vi "Main - Hover.vi"() -> ()   [LabVIEW 2017]
doc: "The myRIO Project template acquires acceleration data from the onboard accelerometer and displays the changes of acceleration values in a waveform chart."
uses:
  <vilib>/myRIO/Instrument Drivers/Onboard IO/PWM/typedefs/PWM Reference.ctl
  <vilib>/myRIO/Common/Instrument Driver Framework/Utilities/typedefs/myRIO Generic Hardware Reference.ctl
  <vilib>/myRIO/Common/Instrument Driver Framework/Utilities/typedefs/Hardware Version Enum.ctl
  <vilib>/myRIO/Common/Instrument Driver Framework/Utilities/typedefs/myRIO v1.0 Reference.ctl
  <vilib>/myRIO/Common/Instrument Driver Framework/Utilities/typedefs/Generic FPGA Reference.ctl
  <vilib>/myRIO/Common/Instrument Driver Framework/myRIO v1.0/PWM/typedefs/PWM Channels Enum.ctl
  <vilib>/myRIO/Instrument Drivers/Onboard IO/PWM/typedefs/PWM Configuration.ctl
  <vilib>/userdefined/High Color/nirio_resource_hc.ctl
  <vilib>/myRIO/Instrument Drivers/Onboard Devices/Accelerometer/typedefs/Accelerometer Reference.ctl
  <vilib>/myRIO/Common/Instrument Driver Framework/myRIO v1.0/Accelerometer/typedefs/Accelerometer Channels List.ctl
  <vilib>/myRIO/Common/Instrument Driver Framework/myRIO v1.0/Accelerometer/typedefs/Accelerometer Channels Enum.ctl
  <vilib>/myRIO/Common/Instrument Driver Framework/Utilities/vis/Is FPGA Ref Available.vi
  <vilib>/myRIO/Common/Instrument Driver Framework/myRIO v1.0/PWM/vis/myRIO v1.1 Open PWM.vi
  <vilib>/myRIO/Instrument Drivers/Onboard IO/PWM/vis/Set Duty Cycle and Frequency.vi
  <vilib>/myRIO/Common/Instrument Driver Framework/myRIO v1.0/Accelerometer/vis/myRIO v1.1 Open Accelerometer.vi
  <vilib>/myRIO/Instrument Drivers/Onboard Devices/Accelerometer/vis/Read.vi
  <vilib>/myRIO/Common/Instrument Driver Framework/Utilities/vis/Validate Channels.vi
  <vilib>/myRIO/Common/Instrument Driver Framework/myRIO v1.0/PWM/vis/myRIO v1.0 Reserve PWM.vi
  <vilib>/myRIO/Common/Instrument Driver Framework/myRIO v1.0/Accelerometer/vis/myRIO v1.0 Reserve Accelerometer.vi
  <vilib>/myRIO/Common/Instrument Driver Framework/myRIO v1.0/UART/vis/myRIO v1.0 Close UART.vi
  <vilib>/myRIO/Common/Instrument Driver Framework/myRIO v1.0/PWM/vis/myRIO v1.0 Build MUX Configuration PWM.vi
  <vilib>/myRIO/Common/Instrument Driver Framework/myRIO v1.0/Resource Manager/vis/myRIO v1.0 Reserve Channel List.vi
  <vilib>/myRIO/Common/Instrument Driver Framework/myRIO v1.0/Accelerometer/vis/myRIO v1.0 Build MUX Configuration Accelerometer.vi
  <vilib>/myRIO/Common/Instrument Driver Framework/myRIO v1.0/Resource Manager/vis/myRIO v1.0 Create Configuration List.vi
  <vilib>/myRIO/Common/Instrument Driver Framework/myRIO v1.0/Resource Manager/vis/myRIO v1.0 Reserve Channel.vi
  <vilib>/myRIO/Common/Instrument Driver Framework/myRIO v1.0/Resource Manager/vis/myRIO v1.0 Unreserve Channel.vi
  <vilib>/myRIO/Common/Instrument Driver Framework/myRIO v1.0/Resource Manager/vis/myRIO v1.0 Build Mutex Name.vi
  <vilib>/Utility/VariantDataType/GetNumericInfo.vi
  <vilib>/Utility/error.llb/Error Cluster From Error Code.vi
  <vilib>/myRIO/Common/Instrument Driver Framework/myRIO v1.0/myRIO v1.1 Open.vi
  <vilib>/myRIO/Common/Instrument Driver Framework/Utilities/vis/IO Manager.vi
  <vilib>/myRIO/Common/Instrument Driver Framework/Utilities/vis/Configuration Manager.vi
  <vilib>/myRIO/Common/Instrument Driver Framework/myRIO v1.0/Resource Manager/vis/myRIO v1.0 Configure IO.vi
  <vilib>/myRIO/Common/Instrument Driver Framework/myRIO v1.0/myRIO v1.0 Close.vi
  <vilib>/myRIO/Common/Instrument Driver Framework/myRIO v1.0/PWM/vis/myRIO v1.0 Write PWM.vi
  <vilib>/myRIO/Common/Instrument Driver Framework/myRIO v1.0/Accelerometer/vis/myRIO v1.0 Get Scaling Constant Accelerometer.vi
  <vilib>/myRIO/Common/Instrument Driver Framework/myRIO v1.0/Accelerometer/vis/myRIO v1.0 Read Accelerometer.vi
  <vilib>/myRIO/Common/Instrument Driver Framework/Utilities/vis/FPGA Ref Manager.vi
  <vilib>/myRIO/Common/Instrument Driver Framework/myRIO v1.0/myRIO v1.0 Reset FPGA.vi
  <vilib>/myRIO/Common/Instrument Driver Framework/myRIO v1.0/IRQ/vis/myRIO v1.0 IRQ Info FGV.vi
  <vilib>/myRIO/Common/Instrument Driver Framework/myRIO v1.0/IRQ/vis/myRIO v1.0 Timer IRQ Info FGV.vi
  <vilib>/myRIO/Common/Instrument Driver Framework/myRIO v1.0/IRQ/vis/myRIO v1.0 ISR Agent.vi
  <vilib>/myRIO/Express VI/Onboard IO/PWM/PWM Express VI.xnode
  <vilib>/myRIO/Instrument Drivers/Onboard IO/PWM/vis/myRIO PWM Open.xnode
  <vilib>/myRIO/Express VI/Onboard Devices/Accelerometer/Accelerometer Express VI.xnode
  <vilib>/myRIO/Instrument Drivers/Onboard Devices/Accelerometer/vis/myRIO Accelerometer Open.xnode
  <vilib>/myRIO/Instrument Drivers/Utilities/Utilities.lvlib
  <vilib>/myRIO/Instrument Drivers/Onboard Devices/Accelerometer/Accelerometer.lvlib
  <vilib>/myRIO/Instrument Drivers/Onboard IO/PWM/PWM.lvlib
panel:
  in  "[ESC]":bool
  out "X rot rate":i16
  out "Y rot rate":i16
  out "Z rot rate":i16
  out "Angular rate [LSB/sec]":cluster{dbl, dbl, dbl}(graph)
  out "Angular displacement [LSB]":T1(graph)
  out "X displacement":dbl format="%#_5g"
  out "Y displacement":dbl format="%#_5g"
  out "Z displacement":dbl format="%#_5g"
  in  "reset integrator":bool
  out "X acc":i16
  out "Y acc":i16
  out "Z acc":i16
  out "Temp":i16
  out "Linear Acceleration [LSB/sec^2]":cluster{i16, i16, i16}(graph)
  in  "Duty Cycle MCC2 : Faixa de operação":dbl
  out "Acceleration 2":T2(graph)
  in  "Brushless controller Duty Cycle":dbl(slide)=0.05 scale=0.05..0.1 scale format="%#_6f"
  in  "Controle sentido M2":bool
  in  "Duty Cycle MCC1 : Faixa de operação":dbl
  in  "Ligar (StandBy)":bool
  in  "Controle sentido M1":bool
  in  "Stop":bool
  # "Overview: The myRIO Project template acquires acceleration data from the onboard accelerometer and displays the changes of acceleration values in a waveform chart.\nInstructions:\n1. Check the myRIO target IP address in the project and make sure the target IP address is correct. \n2. Run this VI."
  # "2"
  # "1"
  # "2"
  # "1"
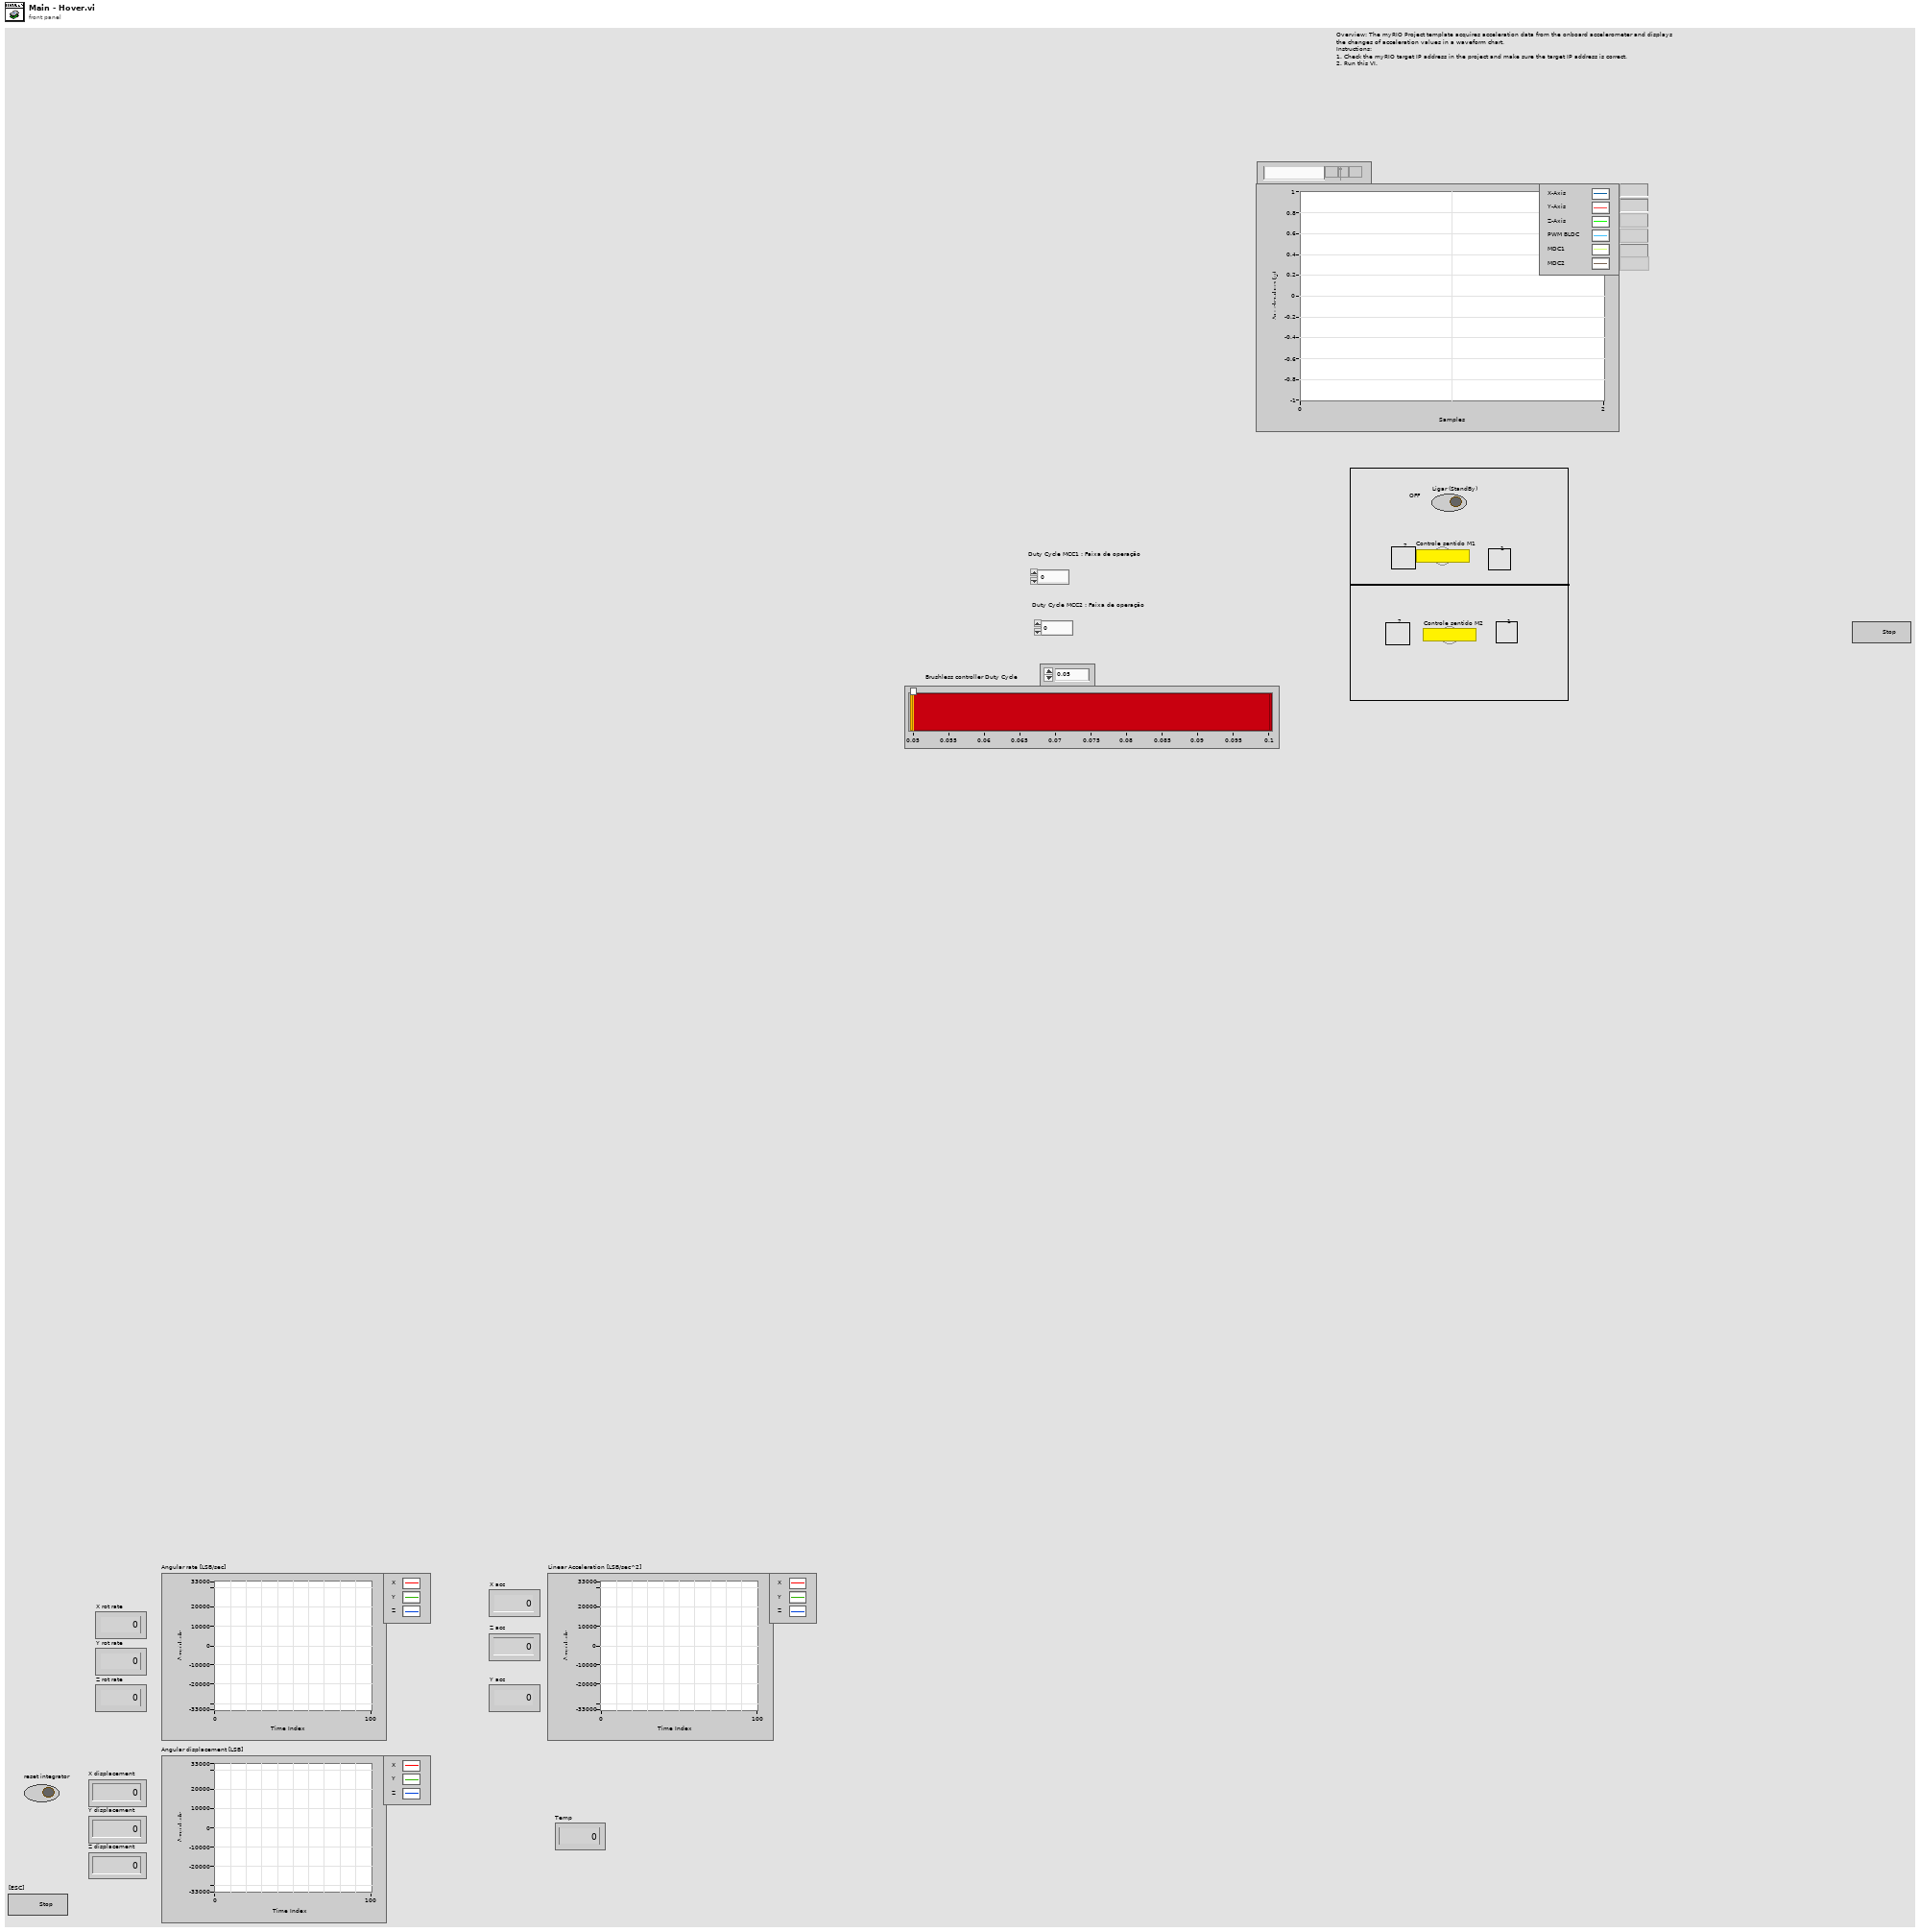
[diagram p1: front panel]
types:
  T1 = cluster{"integral x(t)":dbl, "integral x(t)":dbl, "integral x(t)":dbl}
  T2 = cluster{"X-Axis":dbl, "Y-Axis":dbl, "Z-Axis":dbl, "Brushless controller Duty Cycle":dbl, "\nDuty Cycle MCC1 : Faixa de operação":dbl, "\nDuty Cycle MCC2 : Faixa de operação ":dbl}
  T3 = typedef "PWM.lvlib/PWM Reference.ctl" = cluster{"myRIO Reference":T4, "PWM Channels Enum":T8, "PWM Configuration":T9}
  T4 = typedef "myRIO Generic Hardware Reference.ctl" = cluster{"myRIO Model":T5, "myRIO Hardware Reference":T6}
  T5 = typedef "Hardware Version Enum.ctl" = enum16{"Unknown", "myRIO-1900", "myRIO-1950", "roboRIO", "NI ELVIS RIO CM"}
  T6 = typedef "myRIO v1.0 Reference.ctl" = cluster{"Generic FPGA Reference":T7, "Allow multiple opens":bool}
  T7 = typedef "Generic FPGA Reference.ctl" = refnum<k20>
  T8 = typedef "PWM Channels Enum.ctl" = enum16{"Not Connected", "C/PWM0", "C/PWM1", "A/PWM0", "A/PWM1", "A/PWM2", "B/PWM0", "B/PWM1", "B/PWM2", "PWM/PWM0", "PWM/PWM1", "PWM/PWM2", "PWM/PWM3", "PWM/PWM4", "PWM/PWM5", "PWM/PWM6", "PWM/PWM7", "PWM/PWM8", "PWM/PWM9"}
  T9 = typedef "PWM.lvlib/PWM Configuration.ctl" = cluster{"Frequency":dbl, "Duty Cycle":dbl}
  T10 = typedef "nirio_resource_hc.ctl" = tag
  T11 = typedef "Accelerometer.lvlib/Accelerometer Reference.ctl" = cluster{"myRIO Reference":T4, "Accelerometer Channels List":T12, "LSB Weight":dbl}
  T12 = typedef "Accelerometer Channels List.ctl" = T13[]
  T13 = typedef "Accelerometer Channels Enum.ctl" = enum16{"Not Connected", "X-Axis", "Y-Axis", "Z-Axis"}
  T14 = cluster{"X-Axis":dbl, "Y-Axis":dbl, "Z-Axis":dbl, "Brushless controller Duty Cycle":dbl, "\nDuty Cycle MCC1 : Faixa de operação out":dbl, "\nDuty Cycle MCC2 : Faixa de operação  out":dbl}
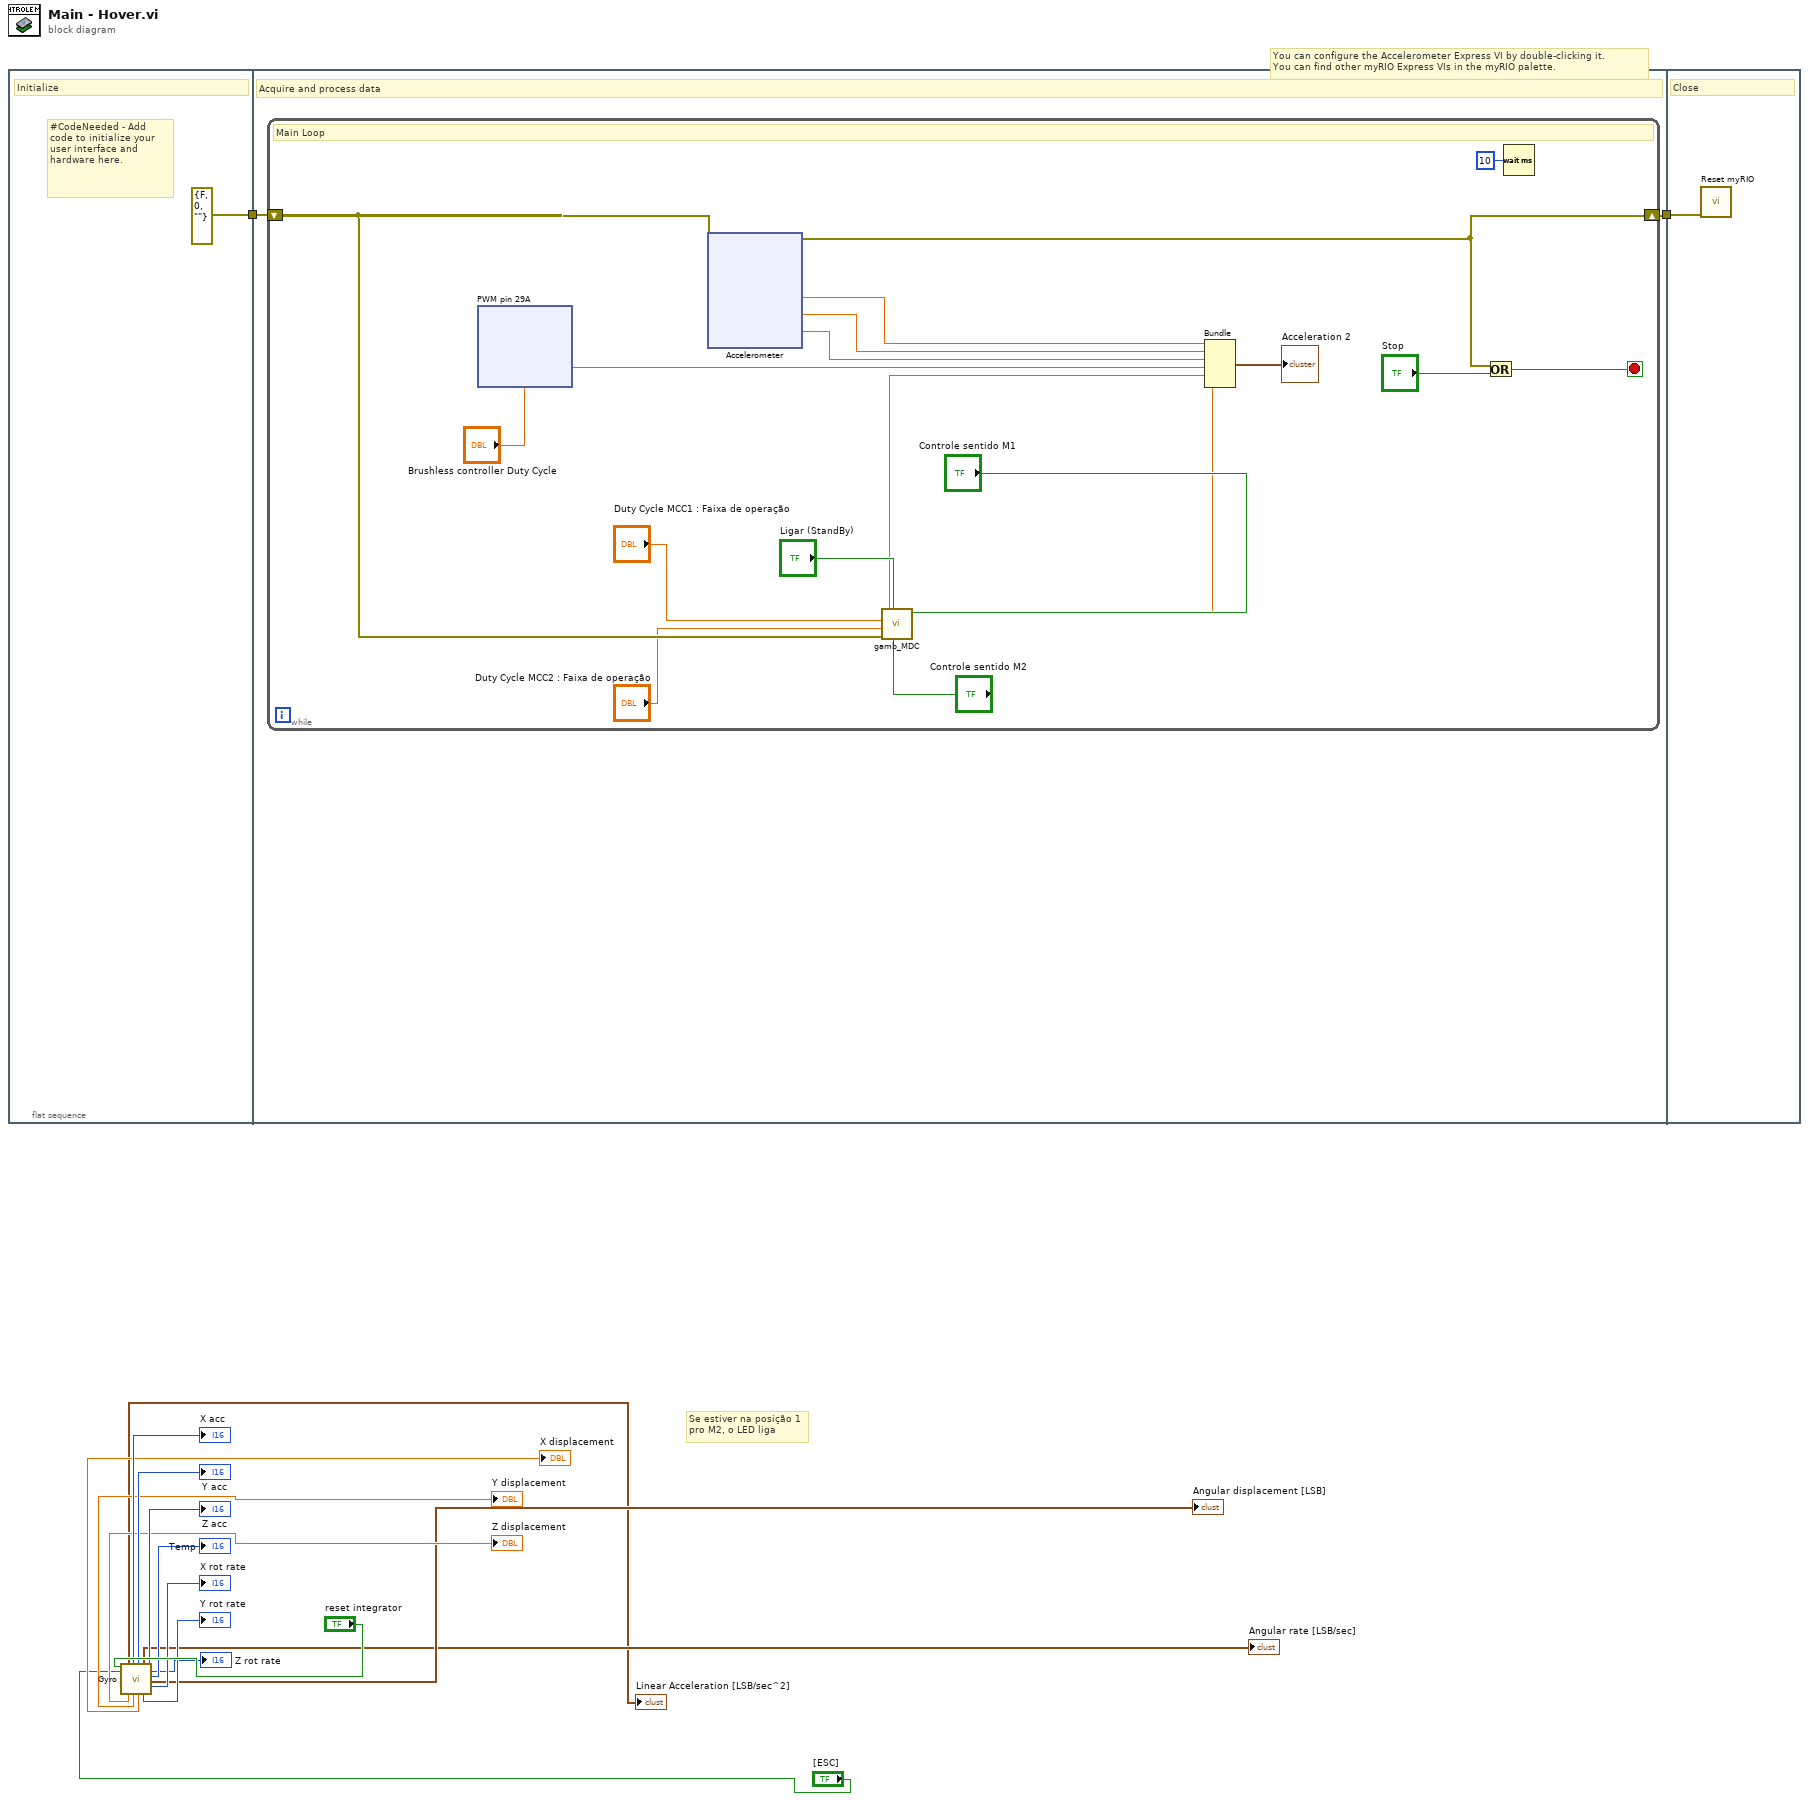
[diagram p0: block diagram]
diagram:
  # "Se estiver na posição 1\npro M2, o LED liga"
  # "You can configure the Accelerometer Express VI by double-clicking it.\nYou can find other myRIO Express VIs in the myRIO palette."
  n1 = flat-sequence {
    tunnel: [errorcluster {"status"=FALSE, "code"=0, "source"=""} ("error in (no error)")] -> w17
    tunnel: w17 -> [w20]
    tunnel: [w19] -> w16
    tunnel: w16 -> [w112]
    frame #0 {
      # "#CodeNeeded - Add code to initialize your user interface and hardware here."
      # "Initialize"
    }
    frame #1 {
      # "Acquire and process data"
      n2 = while {
        shift-right: [w34] -> w19
        shift-left: w20 -> [w30]
        stop <- w36 stop-if-true
        # "Main Loop"
        n3 = xnode "PWM pin 29A"("Duty Cycle"="Brushless controller Duty Cycle") -> ()  [unwired: 1 in, 1 out]
        n4 = xnode "Accelerometer"("error in (no error)"=w30) -> ("X-Axis"=w29:dbl, "Y-Axis"=w28:dbl, "Z-Axis"=w27:dbl, "error out"=w34:errorcluster)
        n5 = call "gamb_MDC.vi"("Controle sentido M2"="Controle sentido M2", "Ligar (StandBy)"="Ligar (StandBy)", "error in (no error)"=w30, "Duty Cycle MCC2 : Faixa de operação  in"="Duty Cycle MCC2 : Faixa de operação", "Duty Cycle MCC1 : Faixa de operação in"="Duty Cycle MCC1 : Faixa de operação", "Controle sentido M1"="Controle sentido M1") -> ("Duty Cycle MCC1 : Faixa de operação out"=w25:dbl, "Duty Cycle MCC2 : Faixa de operação  out"=w23:dbl)  [unwired: 4 in]
        n6 = Bundle("X-Axis"=w29, "Y-Axis"=w28, "Z-Axis"=w27, "Brushless controller Duty Cycle"="Brushless controller Duty Cycle", "Duty Cycle MCC1 : Faixa de operação out"=w25, "Duty Cycle MCC2 : Faixa de operação  out"=w23) -> (→"Acceleration 2":T14)  [unwired: 1 in]
        n7 = Or(x=w34, y="Stop") -> (x .or. y?=w36:bool)
        n8 = Wait (ms)(milliseconds to wait=u32 10) -> ()  [unwired: 1 out]
      }
    }
    frame #2 {
      # "Close"
      n9 = call <vilib>:"Reset myRIO.vi"("error in (no error)"=w112) -> ()  [unwired: 10 in, 1 out]
    }
  }
  n10 = call "Gyro.vi"("reset integrator"="reset integrator", "[ESC]"="[ESC]") -> ("Linear Acceleration [LSB/sec^2]"=→"Linear Acceleration [LSB/sec^2]":cluster{i16, i16, i16}, "Z displacement"=→"Z displacement":dbl, "X acc"=→"X acc":i16, "Y displacement"=→"Y displacement":dbl, "Y acc"=→"Y acc":i16, "X displacement"=→"X displacement":dbl, "Angular rate [LSB/sec]"=→"Angular rate [LSB/sec]":cluster{dbl, dbl, dbl}, "Y rot rate"=→"Y rot rate":i16, "Z acc"=→"Z acc":i16, "Z rot rate"=→"Z rot rate":i16, "Temp"=→"Temp":i16, "Angular displacement [LSB]"=→"Angular displacement [LSB]":T1, "X rot rate"=→"X rot rate":i16)  [unwired: 5 in]
